vi "LINX - Custom commands.vi"() -> ()   [LabVIEW 2019]
uses:
  <vilib>/MakerHub/LINX/Public/Utilities/Open Serial.vi
  <vilib>/MakerHub/LINX/LMH-LINX.lvlib
  vi.lib/LINXx/LINXx.lvlib
panel:
  in  "run swell":bool
  in  "Swell time [ms]":u16
  out "Waveform Graph":u8[](graph)
  in  "stop":bool
  out "Loop Rate (Hz)":u32
  in  "Serial Port":refnum<visa-resource-name>="N/A"
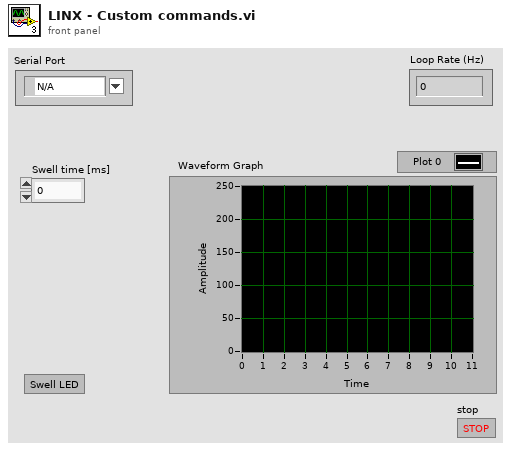
[diagram p1: front panel]
types:
  T1 = typedef "LMH-LINX.lvlib/LINX Ref.ctl" = cluster{"IO":T2, "Interface":T3, "LINX Device Config":T4}
  T2 = typedef "LMH-LINX.lvlib/Platform.ctl" = enum16{"Remote", "Local"}
  T3 = typedef "LMH-LINX.lvlib/Interface.ctl" = enum16{"Serial", "TCP"}
  T4 = typedef "LMH-LINX.lvlib/Device.lvlib/LINX Device Config.ctl" = cluster{"Interface":T3, "COM Port":refnum<visa-resource-name>, "TCP Configuration":T5, "Device Family":u8, "Device ID":u8, "Device Name":string, "TCP Ref":refnum<k5>, "Channels":T6}
  T5 = typedef "LMH-LINX.lvlib/Device.lvlib/TCP Config.ctl" = cluster{"IP Address":string, "Port":u16}
  T6 = typedef "LMH-LINX.lvlib/Channels.ctl" = cluster{"DI":u8[], "DO":u8[], "AI":u8[], "AO":u8[], "PWM":u8[], "QE":u8[], "UART":u8[], "I2C 2":u8[], "SPI":u8[], "CAN":u8[], "Servo":u8[], "AI Ref (V)":dbl, "AI Resolution (Bits)":u8, "AO Ref (V)":dbl, "AO Resolution (Bits)":u8}
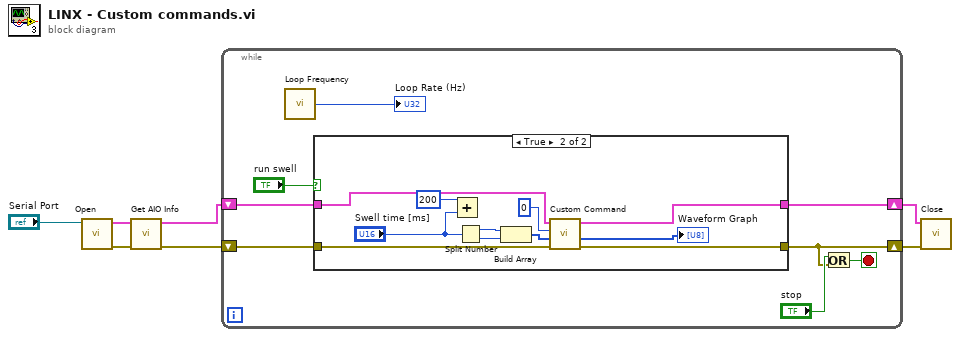
[diagram p0: block diagram]
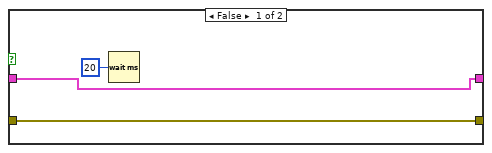
[diagram p2: hidden frame]
diagram:
  n1 = call-poly <vilib>:"Open.vi"("Serial Port"="Serial Port") -> ("Error Out"=w6:errorcluster, "LINX Resource"=w5:T1)  [unwired: 8 in, 1 out]
  n2 = call "Get AIO Info.vi"("Error In"=w6, "LINX Resource"=w5) -> ("Error Out"=w3:errorcluster, "LINX resource"=w4:T1)  [unwired: 6 in, 2 out]
  n3 = while {
    shift-right: [w9] -> w1
    shift-left: w4 -> [w12]
    shift-right: [w10] -> w2
    shift-left: w3 -> [w11]
    stop <- w14 stop-if-true
    n4 = call <vilib>:"Loop Frequency.vi"() -> ("Loop Rate (Hz)"=→"Loop Rate (Hz)":u32)
    n5 = case shown="True" "run swell" {
      tunnel: w12 -> [w16 w29]
      tunnel: w11 -> [w17 w28]
      tunnel: [w17 w27] -> w10
      tunnel: [w16 w26] -> w9
      frame False {
        n6 = Wait (ms)(milliseconds to wait=u32 20) -> ()  [unwired: 1 out]
      }
      frame True {
        n7 = Add(x=u16 200, y="Swell time [ms]") -> ()  [unwired: 1 out]
        n8 = Split Number(x="Swell time [ms]") -> (hi(x)=w24:u8, lo(x)=w23:u8)
        n9 = Build Array(w24, w23) -> (w22:u8[])
        n10 = call <vilib>:"Custom Command.vi"("Error In"=w28, "Data"=w22, "Custom Command Number"=u16 0, "LINX Resource"=w29) -> ("Error Out"=w27:errorcluster, "Response"=→"Waveform Graph":u8[], "LINX Resource"=w26:T1)  [unwired: 4 in, 1 out]
      }
    }
    n11 = Or(x="stop", y=w10) -> (x .or. y?=w14:bool)
  }
  n12 = call <vilib>:"Close.vi"("Error In"=w2, "LINX Resource"=w1) -> ()  [unwired: 9 in, 1 out]
